vi "DBConnector.vi"() -> ()   [LabVIEW 2018]
uses:
  <vilib>/Utility/config.llb/Read Key (Path).vi
  <vilib>/Utility/config.llb/Read Key (String).vi
  <vilib>/addons/database/Connection.llb/DB Tools Open Connec (Path).vi
  <vilib>/addons/database/_DB Variant To Data/Database Variant To Data.xnode
  <vilib>/addons/database/NI_Database_API.lvlib
  <vilib>/Utility/config.llb/NI_LVConfig.lvlib
panel:
  out "Part Amps":dbl format="%.2g"
  out "Part Volts":dbl
  in  "Part Selector":string(combo)
  in  "Config File Path":path
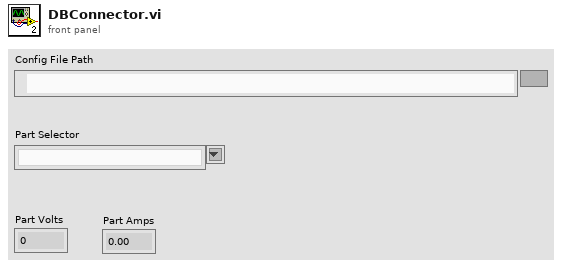
[diagram p1: front panel]
types:
  T1 = typedef "NI_LVConfig.lvlib/Config Data RefNum.ctl" = refnum<k1>
  T2 = typedef "NI_Database_API.lvlib/Conn ObjectReference.ctl" = refnum<k1>
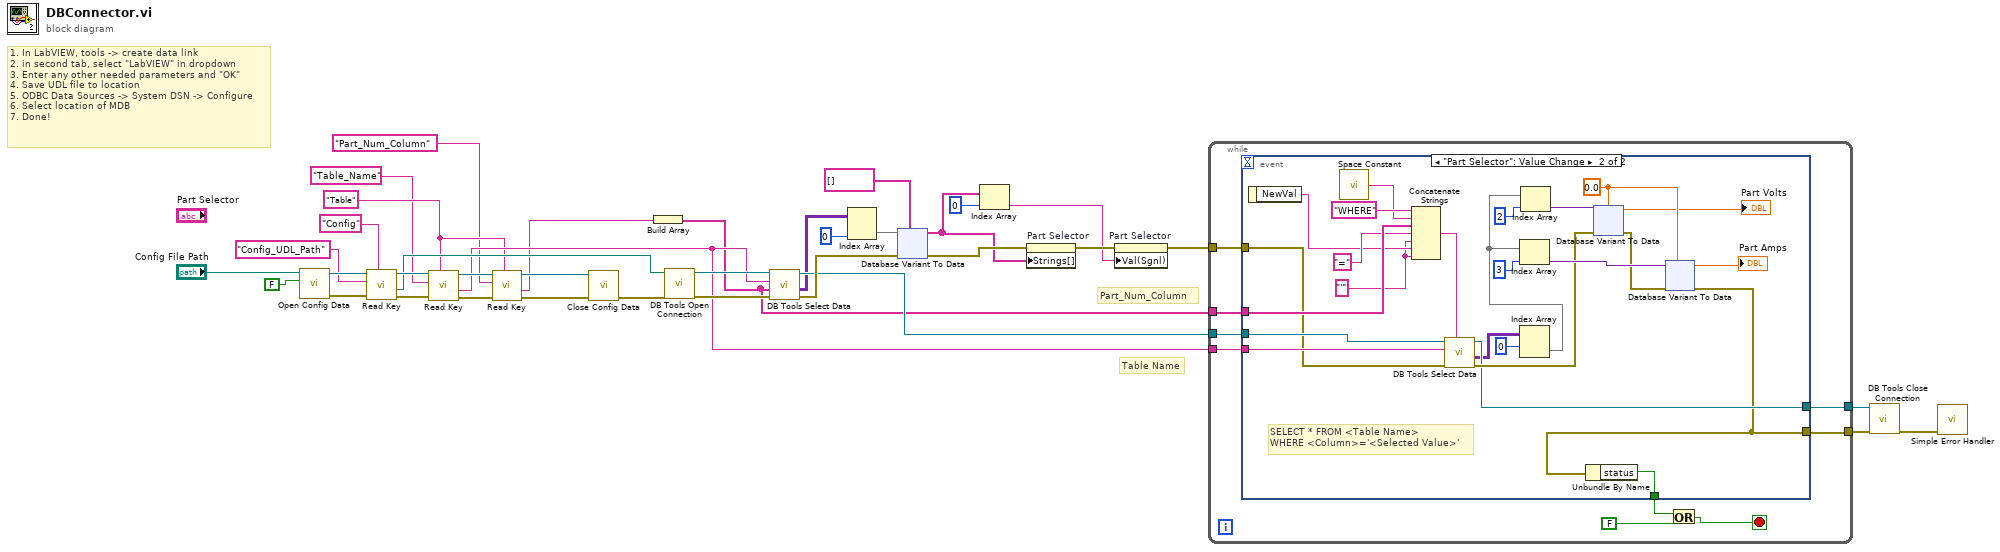
[diagram p0: block diagram]
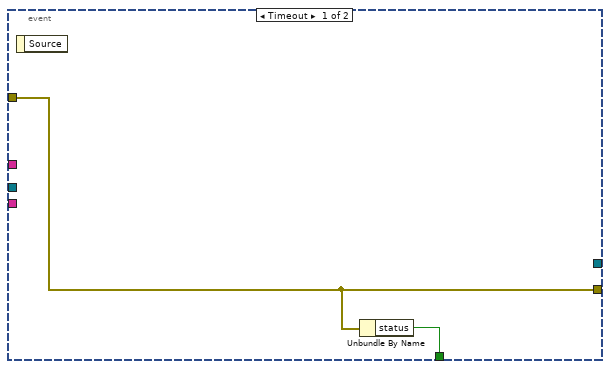
[diagram p2: hidden frame]
diagram:
  w13 = "Table"
  # "1. In LabVIEW, tools -> create data link\n2. in second tab, select \"LabVIEW\" in dropdown\n3. Enter any other needed parameters and \"OK\"\n4. Save UDL file to location\n5. ODBC Data Sources -> System DSN -> Configure\n6. Select location of MDB\n7. Done!"
  # "Part_Num_Column"
  # "Table Name"
  n1 = call <vilib>:"Open Config Data.vi"("create file if necessary (T)"=FALSE, "configuration file path"="Config File Path") -> ("error out"=w34:errorcluster, "refnum"=w35:T1)  [unwired: 7 in, 1 out]
  n2 = call-poly <vilib>:"Read Key.vi"("section"="Config", "error in (no error)"=w34, "key"="Config_UDL_Path", "refnum"=w35) -> ("error out"=w30:errorcluster, "value"=w28:path, "refnum out"=w29:T1)  [unwired: 4 in, 1 out]
  n3 = call-poly <vilib>:"Read Key.vi"("section"=w13, "error in (no error)"=w30, "key"="Table_Name", "refnum"=w29) -> ("error out"=w24:errorcluster, "value"=w18:string, "refnum out"=w25:T1)  [unwired: 4 in, 1 out]
  n4 = call-poly <vilib>:"Read Key.vi"("section"=w13, "error in (no error)"=w24, "key"="Part_Num_Column", "refnum"=w25) -> ("error out"=w22:errorcluster, "value"=w17:string, "refnum out"=w23:T1)  [unwired: 4 in, 1 out]
  n5 = call <vilib>:"Close Config Data.vi"("error in (no error)"=w22, "refnum"=w23) -> ("error out"=w32:errorcluster)  [unwired: 8 in, 1 out]
  n6 = Build Array(w17) -> (w15:string[])
  n7 = call-poly <vilib>:"DB Tools Open Connection.vi"("error in (no error)"=w32, "connection information"=w28) -> ("error out"=w26:errorcluster, "connection reference"=w27:T2)  [unwired: 6 in]
  n8 = call <vilib>:"DB Tools Select Data.vi"("error in (no error)"=w26, "columns"=w15, "table"=w18, "connection reference"=w27) -> ("error out"=w21:errorcluster, "data"=w8:variant[][], "connection reference out"=w16:T2)  [unwired: 2 in]
  n9 = Index Array(array=w8, index (col)=0) -> (element=w7:variant[])  [unwired: 1 in]
  n10 = xnode "Database Variant To Data"("database variant"=w7, "error in (no error)"=w21, "type"=string[] []) -> ("data"=w4:string[], "error out"=w9:errorcluster)
  n11 = Index Array(array=w4, index=0) -> (element=w1:string)
  n12 = property on="Part Selector" class="CmbBox"(error in=w9, "Strings[]"=w4) -> (error out=w2:errorcluster)  [unwired: 1 in, 1 out]
  n13 = property on="Part Selector" class="CmbBox"(error in=w2, "Val(Sgnl)"=w1) -> (error out=w3:errorcluster)  [unwired: 1 in, 1 out]
  n14 = while {
    tunnel: w3 -> [w46]
    tunnel: [w45] -> w19
    tunnel: w18 -> [w42]
    tunnel: w16 -> [w41]
    tunnel: w15 -> [w40]
    tunnel: [w39] -> w14
    stop <- w44 stop-if-true
    n15 = event shown="[1] \"Part Selector\": Value Change" {
      selector: _ -> [_ _]
      dyn-events: _ -> [_ _]
      timeout: _ -> [_ _]
      tunnel: w46 -> [w48 w66]
      tunnel: [w48 w57] -> w45
      tunnel: w42 -> [_ w73]
      tunnel: w41 -> [_ w72]
      tunnel: w40 -> [_ w70]
      tunnel: [_ w61] -> w39
      tunnel: [w47 w56] -> w38
      event Timeout {
        n16 = event-data() -> ()  [unwired: 1 in, 1 out]
        n17 = Unbundle By Name(w48) -> ("status"=w47:bool)
      }
      event "Part Selector": Value Change {
        w58 = "'"
        w64 = 0.0
        # "SELECT * FROM <Table Name> \nWHERE <Column>='<Selected Value>'"
        n18 = event-data() -> ("NewVal"=w59:string)  [unwired: 1 in]
        n19 = call <vilib>:"Space Constant.vi"() -> ("String"=w69:string)
        n20 = Concatenate Strings("WHERE", w69, w70, "=", w58, w59, w58) -> (w67:string)
        n21 = call <vilib>:"DB Tools Select Data.vi"("condition"=w67, "error in (no error)"=w66, "table"=w73, "connection reference"=w72) -> ("error out"=w62:errorcluster, "data"=w54:variant[][], "connection reference out"=w61:T2)  [unwired: 2 in]
        n22 = Index Array(array=w54, index (row)=0) -> (element=w53:variant[])  [unwired: 1 in]
        n23 = Index Array(array=w53, index=3) -> (element=w63:variant)
        n24 = Index Array(array=w53, index=2) -> (element=w65:variant)
        n25 = xnode "Database Variant To Data"("database variant"=w65, "error in (no error)"=w62, "type"=w64) -> ("data"=→"Part Volts":dbl, "error out"=w60:errorcluster)
        n26 = xnode "Database Variant To Data"("database variant"=w63, "error in (no error)"=w60, "type"=w64) -> ("data"=→"Part Amps":dbl, "error out"=w57:errorcluster)
        n27 = Unbundle By Name(w57) -> ("status"=w56:bool)
      }
    }
    n28 = Or(x=w38, y=FALSE) -> (x .or. y?=w44:bool)
  }
  n29 = call <vilib>:"DB Tools Close Connection.vi"("error in (no error)"=w19, "connection reference"=w14) -> ("error out"=w31:errorcluster)  [unwired: 5 in]
  n30 = call <vilib>:"Simple Error Handler.vi"("error in (no error)"=w31) -> ()  [unwired: 4 in, 5 out]
